vi "条件结构的使用.vi"() -> ()   [LabVIEW 2018]
panel:
  out "最大值":dbl
  out "数值4":dbl
  out "数值3":dbl
  out "数值2":dbl
  out "数值1":dbl
  # "实验内容：创建一个VI，比较四个数，输出最大值。\n\n实验设备：电脑、Labview软件\n\n实验步骤：编写比较四个数的条件结构程序，不断调试，得到预期结果，并进行记录。"
  # "20174080221\n王靖\n电子二班"
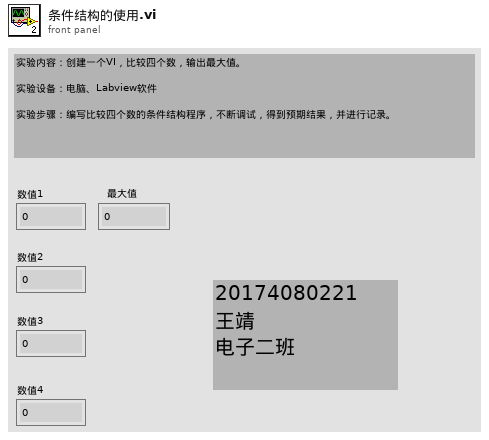
[diagram p1: front panel]
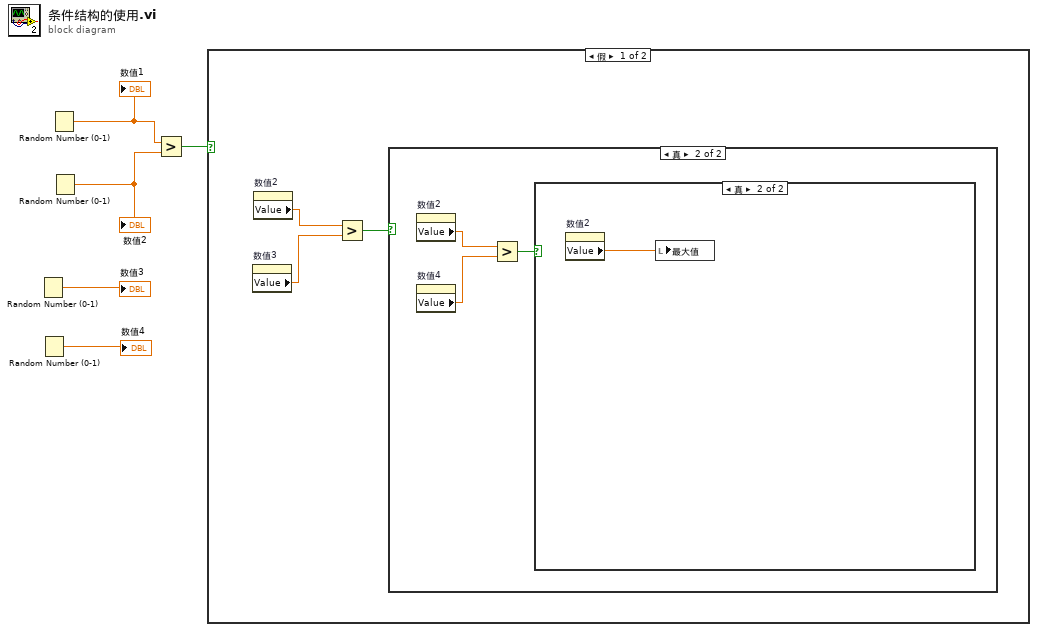
[diagram p0: block diagram]
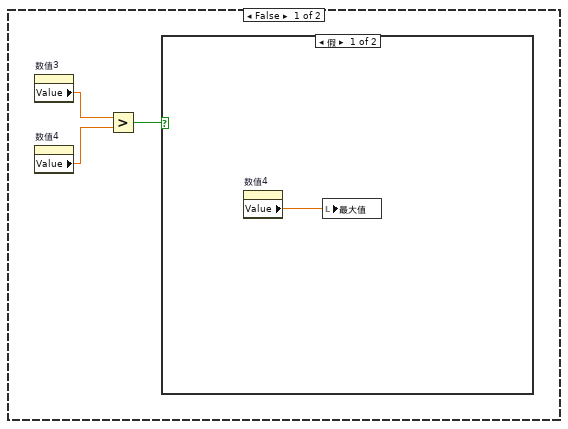
[diagram p2: hidden frame]
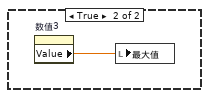
[diagram p3: hidden frame]
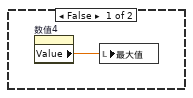
[diagram p4: hidden frame]
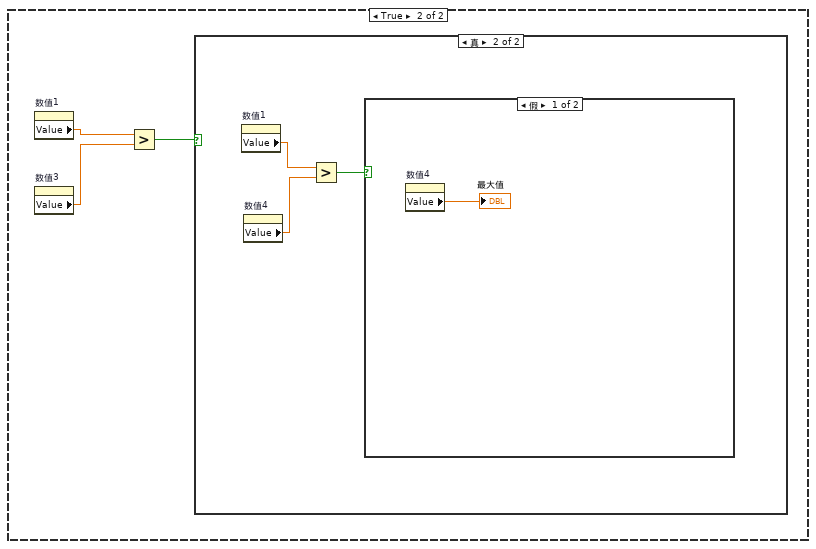
[diagram p5: hidden frame]
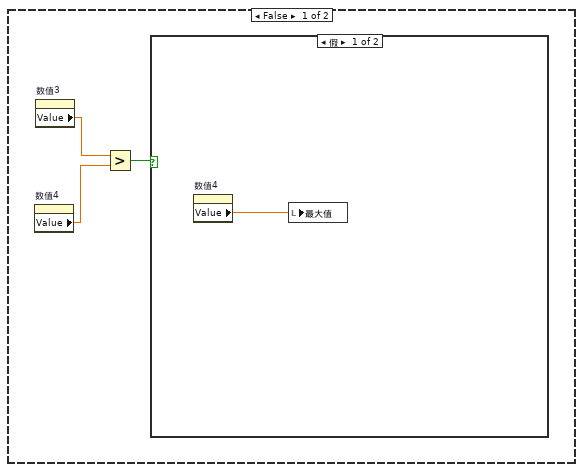
[diagram p6: hidden frame]
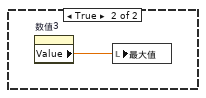
[diagram p7: hidden frame]
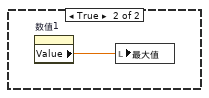
[diagram p8: hidden frame]
diagram:
  n1 = Random Number (0-1)() -> (number: 0 to 1=→"数值3":dbl)
  n2 = Random Number (0-1)() -> (number: 0 to 1=→"数值4":dbl)
  n3 = Random Number (0-1)() -> (number: 0 to 1=w5:dbl)
  "数值1" <- w5
  n4 = Random Number (0-1)() -> (number: 0 to 1=w4:dbl)
  "数值2" <- w4
  n5 = Greater?(x=w5, y=w4) -> (0:w3:bool)
  n6 = case shown="假" w3 {
    frame False {
      n7 = property on="数值3" class="DigNum (严格)"() -> ("Value"=w7:dbl)  [unwired: 2 in, 2 out]
      n8 = property on="数值2" class="DigNum (严格)"() -> ("Value"=w8:dbl)  [unwired: 2 in, 2 out]
      n9 = Greater?(x=w8, y=w7) -> (0:w6:bool)
      n10 = case shown="真" w6 {
        frame False {
          n11 = property on="数值3" class="DigNum (严格)"() -> ("Value"=w11:dbl)  [unwired: 2 in, 2 out]
          n12 = property on="数值4" class="DigNum (严格)"() -> ("Value"=w10:dbl)  [unwired: 2 in, 2 out]
          n13 = Greater?(x=w11, y=w10) -> (0:w9:bool)
          n14 = case shown="假" w9 {
            frame False {
              n15 = property on="数值4" class="DigNum (严格)"() -> ("Value"=w12:dbl)  [unwired: 2 in, 2 out]
              n16 = local write "最大值"(w12) -> ()
            }
            frame True {
              n17 = property on="数值3" class="DigNum (严格)"() -> ("Value"=w13:dbl)  [unwired: 2 in, 2 out]
              n18 = local write "最大值"(w13) -> ()
            }
          }
        }
        frame True {
          n19 = property on="数值2" class="DigNum (严格)"() -> ("Value"=w16:dbl)  [unwired: 2 in, 2 out]
          n20 = property on="数值4" class="DigNum (严格)"() -> ("Value"=w15:dbl)  [unwired: 2 in, 2 out]
          n21 = Greater?(x=w16, y=w15) -> (0:w14:bool)
          n22 = case shown="真" w14 {
            frame False {
              n23 = property on="数值4" class="DigNum (严格)"() -> ("Value"=w17:dbl)  [unwired: 2 in, 2 out]
              n24 = local write "最大值"(w17) -> ()
            }
            frame True {
              n25 = property on="数值2" class="DigNum (严格)"() -> ("Value"=w18:dbl)  [unwired: 2 in, 2 out]
              n26 = local write "最大值"(w18) -> ()
            }
          }
        }
      }
    }
    frame True {
      n27 = property on="数值1" class="DigNum (严格)"() -> ("Value"=w21:dbl)  [unwired: 2 in, 2 out]
      n28 = property on="数值3" class="DigNum (严格)"() -> ("Value"=w20:dbl)  [unwired: 2 in, 2 out]
      n29 = Greater?(x=w21, y=w20) -> (0:w19:bool)
      n30 = case shown="真" w19 {
        frame False {
          n31 = property on="数值4" class="DigNum (严格)"() -> ("Value"=w23:dbl)  [unwired: 2 in, 2 out]
          n32 = property on="数值3" class="DigNum (严格)"() -> ("Value"=w24:dbl)  [unwired: 2 in, 2 out]
          n33 = Greater?(x=w24, y=w23) -> (0:w22:bool)
          n34 = case shown="假" w22 {
            frame False {
              n35 = property on="数值4" class="DigNum (严格)"() -> ("Value"=w25:dbl)  [unwired: 2 in, 2 out]
              n36 = local write "最大值"(w25) -> ()
            }
            frame True {
              n37 = property on="数值3" class="DigNum (严格)"() -> ("Value"=w26:dbl)  [unwired: 2 in, 2 out]
              n38 = local write "最大值"(w26) -> ()
            }
          }
        }
        frame True {
          n39 = property on="数值1" class="DigNum (严格)"() -> ("Value"=w29:dbl)  [unwired: 2 in, 2 out]
          n40 = property on="数值4" class="DigNum (严格)"() -> ("Value"=w28:dbl)  [unwired: 2 in, 2 out]
          n41 = Greater?(x=w29, y=w28) -> (0:w27:bool)
          n42 = case shown="假" w27 {
            frame False {
              n43 = property on="数值4" class="DigNum (严格)"() -> ("Value"=→"最大值":dbl)  [unwired: 2 in, 2 out]
            }
            frame True {
              n44 = property on="数值1" class="DigNum (严格)"() -> ("Value"=w31:dbl)  [unwired: 2 in, 2 out]
              n45 = local write "最大值"(w31) -> ()
            }
          }
        }
      }
    }
  }
